vi "test Extract Signal.vi"(11 "Test Case In":refnum<class "Test PCAN.lvclass">) -> (0 "error out":errorcluster, 3 "Test Case Out":refnum<class "Test PCAN.lvclass">)   [LabVIEW 2023]
uses:
  Devices/CAN Interfaces/PCAN/Tests/Test PCAN.lvclass
  C:/Program Files/National Instruments/LabVIEW 2023/vi.lib/Astemes/LUnit/Test Case.lvclass
  <vilib>/Astemes/LUnit/Test Case.lvclass/Test Case.ctl
  4993e8ee-a06a-463a-9684-69129f64d5ce.vi
  <vilib>/Astemes/LUnit/Append Pass Result.vi
  <vilib>/Astemes/LUnit/Append Fail Result.vi
  <vilib>/Astemes/LUnit/Describe Comparison.vi
  <vilib>/Astemes/LUnit/Compare Variants.vi
  <vilib>/Astemes/LUnit/Run In UI.vi
  <vilib>/Utility/error.llb/Clear Errors.vi
  <vilib>/Astemes/LUnit/Describe Variant.vi
  CAN Frame.lvclass
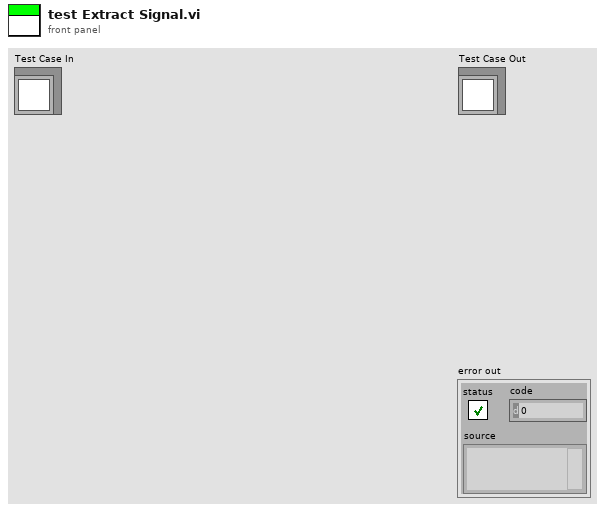
[diagram p1: front panel]
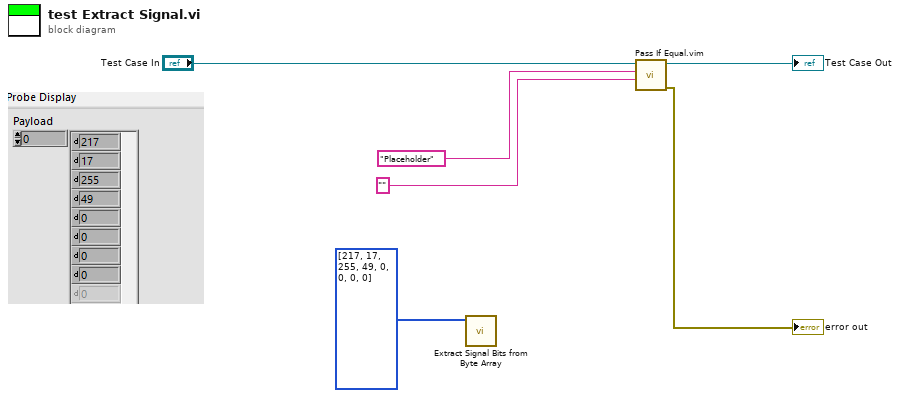
[diagram p0: block diagram]
diagram:
  n1 = call "Extract Signal Bits from Byte Array.vi"("Payload"=u8[] [217, 17, 255, 49, 0, 0, 0, 0]) -> ()  [unwired: 10 in, 1 out]
  n2 = call "Pass If Equal.vim"("Actual"="", "Expected"="Placeholder", "LUnit Test Case In"="Test Case In") -> ("error out"=→"error out":errorcluster, "LUnit Test Case Out"=→"Test Case Out":refnum<class "Test PCAN.lvclass">)  [unwired: 7 in]
